vi "CLASS - Display2DTrain.vi"(8 "error in":errorcluster, 11 "Local":T6) -> (0 "error out":errorcluster, 3 "Local Out":T6)   [LabVIEW 2020]
doc: "Display the 2D graph"
uses:
  Controls/2DParameters.ctl
  _Controls/Datas.ctl
  _Controls/PointPropertyMultipleLabel.ctl
  _Controls/Style.ctl
  _Controls/2DData.ctl
types:
  T1 = typedef "2DParameters.ctl" = cluster{"Plot":refnum<vi>, "Data":T2, "Display":cluster{"Choice":enum16{"All", "Train", "Test"}, "Indexe":cluster{"X":i32, "Y":i32}}, "Property":T3}
  T2 = typedef "Datas.ctl" = cluster{"Split":cluster{"X Train":dbl[][], "X Test":dbl[][], "Y Train":dbl[][], "Y Test":dbl[][]}, "Predict":dbl[][]}
  T3 = typedef "PointPropertyMultipleLabel.ctl" = cluster{"Train Style":T4, "Test OK Style":T4, "Label Color":u32[], "Test NO OK":cluster{"Style":T4, "Color":u32}}
  T4 = typedef "Style.ctl" = enum16{"Empty circle", "Full circle", "Empty square", "Full square", "Cross"}
  T5 = typedef "2DData.ctl" = cluster{"Tag":i32, "X":dbl[], "Y":dbl[]}
  T6 = cluster{"Parameters":T1, "2D Array":cluster{"X":dbl[], "Y":dbl[]}[], "Rating 2D Array":T5[], "Point ID":cluster{"DataUse":enum16{"Dataset", "Train", "Test"}, "Color":u32}[], "GoodPredict":i32}
  T7 = cluster{"DataUse":enum16{"Dataset", "Train", "Test"}, "Color":u32}[]
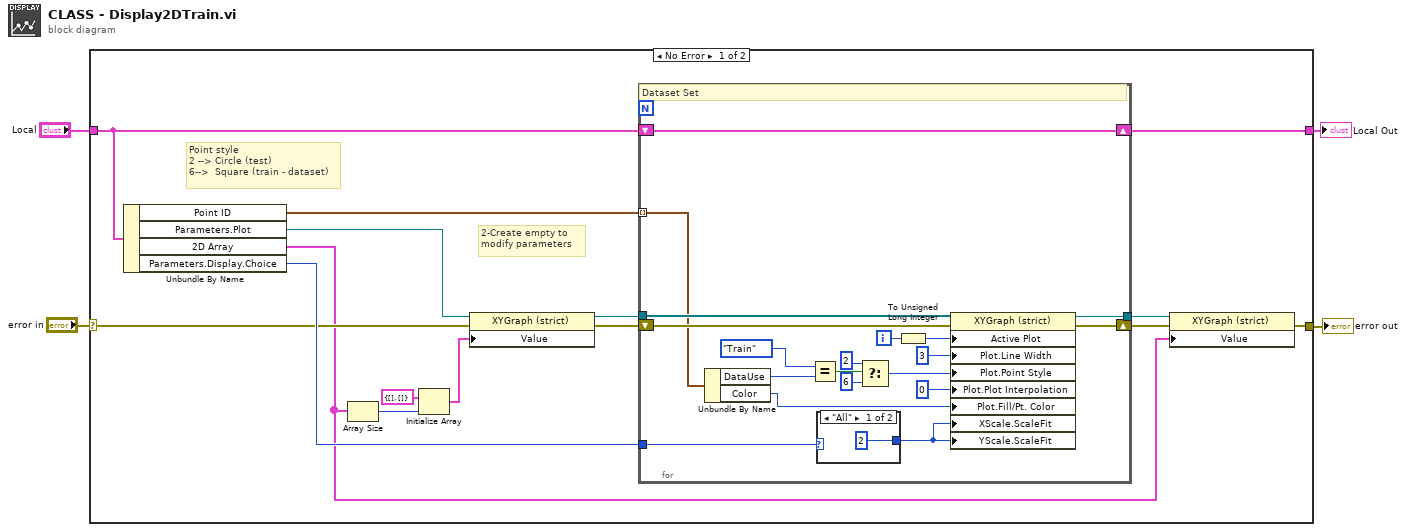
[diagram p0: block diagram]
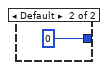
[diagram p2: hidden frame]
diagram:
  n1 = case shown="No Error" "error in" {
    selector: "error in" -> [w8 w42]
    tunnel: "Local" -> [w17 w41]
    tunnel: [w10 w42] -> w4
    tunnel: [w14 w41] -> w1
    frame No Error {
      # "Point style \n2 --> Circle (test)\n6-->  Square (train - dataset)"
      # "2-Create empty to \nmodify parameters"
      n2 = Unbundle By Name(w17) -> ("Point ID"=w7:T7, "Parameters.Plot"=w5:refnum<vi>, "2D Array"=w6:cluster{"X":dbl[], "Y":dbl[]}[], "Parameters.Display.Choice"=w9:enum16{"All", "Train", "Test"})
      n3 = Array Size(array=w6) -> (size(s)=w13:i32)
      n4 = Initialize Array(cluster{dbl[], dbl[]} {[], []}, w13) -> (w18:cluster{dbl[], dbl[]}[])
      n5 = property class="XYGraph (strict)"(reference=w5, error in=w8, "Value"=w18) -> (reference out=w15:refnum<vi>, error out=w16:errorcluster)
      n6 = for {
        tunnel: w15 -> [w38]
        tunnel: w7 -> [w31] mode=indexing
        shift-right: [w25] -> w14
        shift-left: w17 -> [w25]
        tunnel: [w22] -> w12
        shift-right: [w34] -> w11
        shift-left: w16 -> [w37]
        tunnel: w9 -> [w21]
        i -> [w33]
        # "Dataset Set"
        n7 = Unbundle By Name(w31) -> ("DataUse"=w26:enum16{"Dataset", "Train", "Test"}, "Color"=w24:u32)
        n8 = Equal?(x=enum16{"Dataset", "Train", "Test"}."Train", y=w26) -> (x = y?=w30:bool)
        n9 = case shown="\"All\"" w21 {
          tunnel: [u8 2 ("X Scale.Scale Fit") u8 0 ("X Scale.Scale Fit")] -> w20
          frame "All" {
          }
          frame Default {
          }
        }
        n10 = Select(t=u8 2 ("Plot.Point Style"), s=w30, f=u8 6 ("Plot.Point Style")) -> (s? t:f=w27:u8)
        n11 = To Unsigned Long Integer(number=w33) -> (unsigned 32bit integer=w32:u32)
        n12 = property class="XYGraph (strict)"(reference=w38, error in=w37, "Active Plot"=w32, "Plot.Line Width"=u8 3, "Plot.Point Style"=w27, "Plot.Plot Interpolation"=u8 0, "Plot.Fill/Pt. Color"=w24, "XScale.ScaleFit"=w20, "YScale.ScaleFit"=w20) -> (reference out=w22:refnum<vi>, error out=w34:errorcluster)
      }
      n13 = property class="XYGraph (strict)"(reference=w12, error in=w11, "Value"=w6) -> (error out=w10:errorcluster)  [unwired: 1 out]
    }
    frame Error {
    }
  }
  "error out" <- w4
  "Local Out" <- w1
